vi "Scan_1.vi"(4 "error in":errorcluster, 5 "input main cluster":T2, 7 "Map geometry":T1) -> (0 "error out":errorcluster, 1 "output main cluster":T2)   [LabVIEW 2010]
uses:
  Main_cluster.ctl
  <vilib>/vision/Image Controls.llb/IMAQ Image.ctl
  PI E710 Stage.lvlib
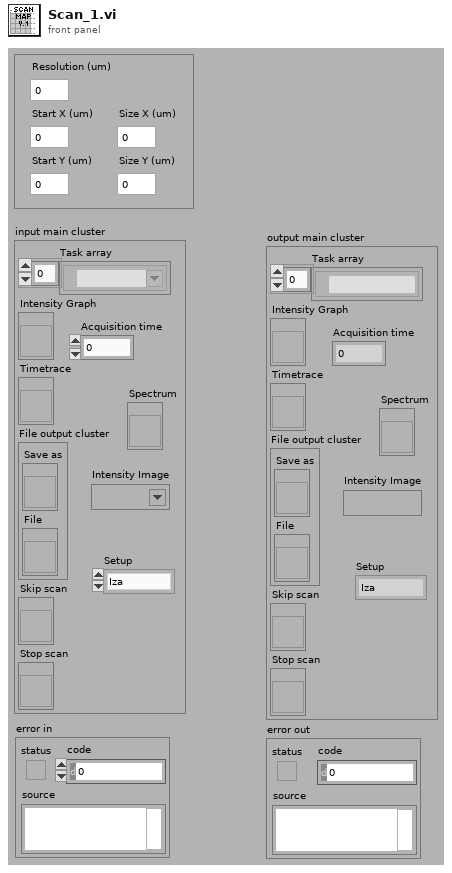
[diagram p1: front panel]
types:
  T1 = cluster{"Size Y (um)":dbl, "Size X (um)":dbl, "Start Y (um)":dbl, "Start X (um)":dbl, "Resolution (um)":dbl}
  T2 = typedef "Main_cluster.ctl" = cluster{"Task array":refnum<k21>[], "Intensity Graph":refnum<vi>, "Timetrace":refnum<vi>, "File output cluster":cluster{"Save as":refnum<vi>, "File":refnum<vi>}, "Skip scan":refnum<vi>, "Stop scan":refnum<vi>, "Acquisition time":dbl, "Setup":enum16{"Iza", "Lukasz"}, "Spectrum":refnum<vi>, "Intensity Image":T3}
  T3 = typedef "IMAQ Image.ctl" = refnum<image>
  T4 = enum16{"open", "replace", "create", "open or create", "replace or create", "replace or create with confirmation"}
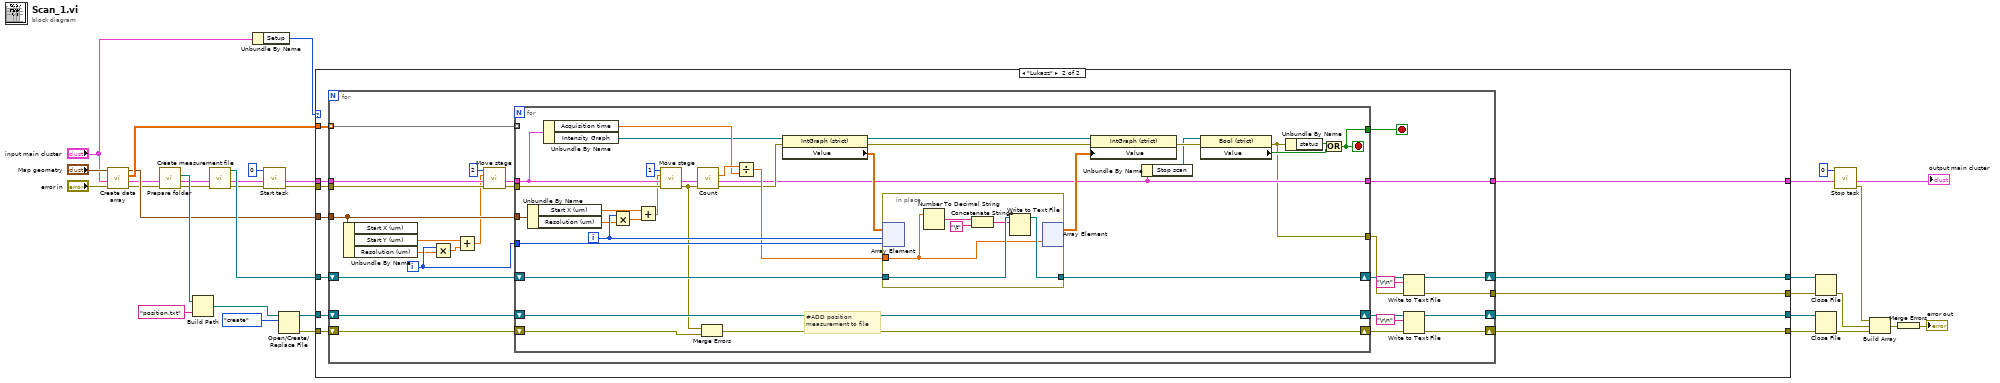
[diagram p0: block diagram]
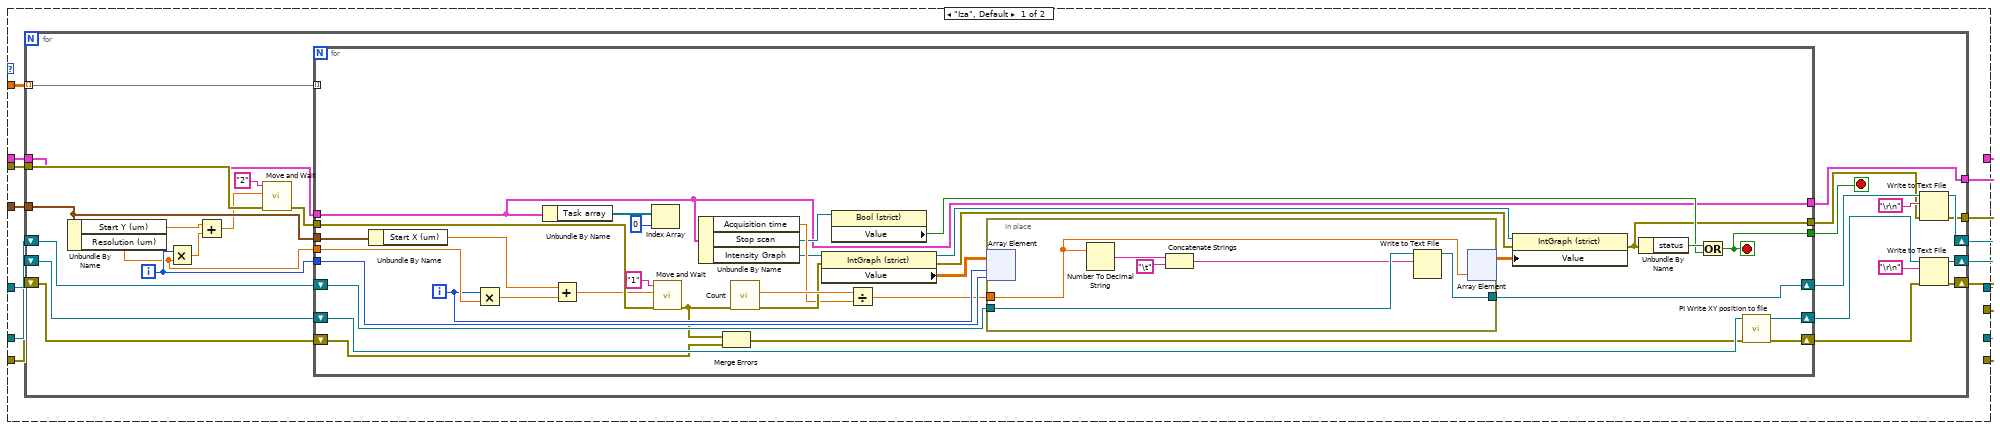
[diagram p2: hidden frame]
diagram:
  n1 = call "Create data array.vi"("error in"="error in", "input main cluster"="input main cluster", "Map geometry"="Map geometry") -> ("error out"=w3:errorcluster, "output main cluster"=w4:T2, "Data array"=w19:dbl[][], "Map geometry out"=w6:T1)  [unwired: 1 in]
  n2 = call "Prepare folder.vi"("error in"=w3, "input main cluster"=w4) -> ("error out"=w8:errorcluster, "output main cluster"=w9:T2, "created path"=w23:path)  [unwired: 3 in]
  n3 = Build Path(base path=w23, name or relative path="position.txt" ("string")) -> (appended path=w30:path)
  n4 = call "Create measurement file.vi"("error in"=w8, "input main cluster"=w9) -> ("error out"=w17:errorcluster, "output main cluster"=w11:T2, "refnum out"=w34:refnum<file>)  [unwired: 3 in]
  n5 = Unbundle By Name("input main cluster") -> ("Setup"=w20:enum16{"Iza", "Lukasz"})
  n6 = call "Start task.vi"("error in"=w17, "input main cluster"=w11, "index"=0) -> ("error out"=w16:errorcluster, "output cluster"=w14:T2)  [unwired: 3 in]
  n7 = Open/Create/Replace File(file path (use dialog)=w30, operation (0:open)=T4."create") -> (refnum out=w29:refnum<file>, error out=w28:errorcluster)  [unwired: 4 in, 1 out]
  n8 = case shown="\"Lukasz\"" w20 {
    tunnel: w16 -> [w46 w124]
    tunnel: w34 -> [w45 w123]
    tunnel: [w44 w122] -> w33
    tunnel: [w43 w121] -> w32
    tunnel: w14 -> [w42 w120]
    tunnel: [w41 w119] -> w18
    tunnel: w19 -> [w40 w118]
    tunnel: w6 -> [w39 w117]
    tunnel: w29 -> [w38 w116]
    tunnel: w28 -> [w37 w115]
    tunnel: [w36 w114] -> w27
    tunnel: [w35 w113] -> w2
    frame "Iza", Default {
      n9 = for {
        tunnel: w46 -> [w72]
        tunnel: [w61] -> w43
        shift-right: [w64] -> w44
        shift-left: w45 -> [w67]
        tunnel: w42 -> [w57]
        tunnel: [w60] -> w41
        tunnel: w39 -> [w58]
        tunnel: w40 -> [w47] mode=indexing
        shift-right: [w52] -> w35
        shift-left: w37 -> [w55]
        shift-right: [w50] -> w36
        shift-left: w38 -> [w56]
        i -> [w68]
        stop <- w66 stop-if-true
        n10 = Unbundle By Name(w58) -> ("Start Y (um)"=w59:dbl, "Resolution (um)"=w48:dbl)
        n11 = Multiply(x=w68, y=w48) -> (x*y=w70:dbl)
        n12 = Add(x=w59, y=w70) -> (x+y=w49:dbl)
        n13 = call "Move and Wait.vi"("error IO"=w72, "Absolute position"=w49, "Axis"="2" ("String")) -> ("error out"=w71:errorcluster)  [unwired: 4 in]
        n14 = for {
          tunnel: [w90] -> w62
          tunnel: w71 -> [w88]
          tunnel: w68 -> [w104]
          tunnel: w48 -> [w102]
          tunnel: [w81] -> w66
          shift-right: [w98] -> w65
          shift-left: w67 -> [w99]
          tunnel: w57 -> [w76]
          tunnel: [w76] -> w60
          tunnel: w58 -> [w85]
          tunnel: w47 -> [_] mode=indexing
          shift-right: [w78] -> w53
          shift-left: w55 -> [w74]
          shift-right: [w79] -> w51
          shift-left: w56 -> [w80]
          i -> [w100]
          stop <- w81 stop-if-true
          n15 = Unbundle By Name(w85) -> ("Start X (um)"=w86:dbl)
          n16 = Multiply(x=w100, y=w102) -> (x*y=w103:dbl)
          n17 = Unbundle By Name(w76) -> ("Task array"=w83:refnum<k21>[])
          n18 = Add(x=w86, y=w103) -> (x+y=w77:dbl)
          n19 = Index Array(array=w83, index=0) -> ()  [unwired: 1 out]
          n20 = call "Move and Wait.vi"("error IO"=w88, "Absolute position"=w77, "Axis"="1" ("String")) -> ("error out"=w73:errorcluster)  [unwired: 4 in]
          n21 = Unbundle By Name(w76) -> ("Acquisition time"=w89:dbl, "Stop scan"=w87:refnum<vi>, "Intensity Graph"=w84:refnum<vi>)
          n22 = Merge Errors(w73, w74) -> (w75:errorcluster)
          n23 = call "Count.vi"("error in"=w73) -> ("error out"=w92:errorcluster, "Counts"=w95:dbl)  [unwired: 4 in, 1 out]
          n24 = property class="IntGraph (strict)"(reference=w84, error in=w92) -> (reference out=w93:refnum<vi>, error out=w91:errorcluster, "Value"=w106:dbl[][])
          n25 = property class="Bool (strict)"(reference=w87) -> ("Value"=w94:bool)  [unwired: 1 in, 2 out]
          n26 = Divide(x=w95, y=w89) -> (x/y=w96:dbl)
          n27 = in-place {
            in-place-border: w96 -> [w109]
            in-place-border: w99 -> [w112]
            in-place-border: [w111] -> w98
            n28 = in-place-array #1(w106, w100, w104) -> ()  [unwired: 1 out]
            n29 = Number To Decimal String(number=w109) -> (decimal integer string=w110:string)  [unwired: 1 in]
            n30 = Concatenate Strings(w110, "\t") -> (w107:string)
            n31 = Write to Text File(file (use dialog)=w112, text=w107) -> (refnum out=w111:refnum<file>)  [unwired: 2 in, 2 out]
            n32 = in-place-array #1(w109) -> (w105:dbl[][])  [unwired: 2 out]
          }
          n33 = property class="IntGraph (strict)"(reference=w93, error in=w91, "Value"=w105) -> (error out=w90:errorcluster)  [unwired: 1 out]
          n34 = Unbundle By Name(w90) -> ("status"=w97:bool)
          n35 = Or(x=w97, y=w94) -> (x .or. y?=w81:bool)
          n36 = call "PI Write XY position to file.vi"("error in"=w75, "refnum in"=w80) -> ("error out"=w78:errorcluster, "refnum out"=w79:refnum<file>)  [unwired: 4 in]
        }
        n37 = Write to Text File(file (use dialog)=w65, text="\r\n", error in=w62) -> (refnum out=w64:refnum<file>, error out=w61:errorcluster)  [unwired: 1 in, 1 out]
        n38 = Write to Text File(file (use dialog)=w51, text="\r\n", error in=w53) -> (refnum out=w50:refnum<file>, error out=w52:errorcluster)  [unwired: 1 in, 1 out]
      }
    }
    frame "Lukasz" {
      n39 = for {
        tunnel: w124 -> [w131]
        tunnel: [w143] -> w121
        shift-right: [w146] -> w122
        shift-left: w123 -> [w149]
        tunnel: w120 -> [w129]
        tunnel: [w142] -> w119
        tunnel: w117 -> [w140]
        tunnel: w118 -> [w139] mode=indexing
        shift-right: [w134] -> w113
        shift-left: w115 -> [w137]
        shift-right: [w132] -> w114
        shift-left: w116 -> [w138]
        i -> [w150]
        stop <- w148 stop-if-true
        n40 = Unbundle By Name(w140) -> ("Start Y (um)"=w141:dbl, "Resolution (um)"=w127:dbl)  [unwired: 1 out]
        n41 = Multiply(x=w150, y=w127) -> (x*y=w151:dbl)
        n42 = Add(x=w141, y=w151) -> (x+y=w125:dbl)
        n43 = call "Move stage.vi"("error in"=w131, "input main cluster"=w129, "position"=w125, "Axis"=2) -> ("error out"=w130:errorcluster, "output main cluster"=w128:T2)  [unwired: 2 in]
        n44 = for {
          tunnel: [w153] -> w144
          tunnel: w130 -> [w161]
          tunnel: w150 -> [w182]
          tunnel: [w166] -> w148
          shift-right: [w178] -> w147
          shift-left: w149 -> [w179]
          tunnel: w128 -> [w160]
          tunnel: [w155] -> w142
          tunnel: w140 -> [w168]
          tunnel: w139 -> [_] mode=indexing
          shift-right: [w164] -> w135
          shift-left: w137 -> [w163]
          shift-right: [w165] -> w133
          shift-left: w138 -> [w165]
          i -> [w180]
          stop <- w166 stop-if-true
          # "#ADD position \nmeasurement to file"
          n45 = Unbundle By Name(w168) -> ("Start X (um)"=w169:dbl, "Resolution (um)"=w159:dbl)
          n46 = Unbundle By Name(w160) -> ("Acquisition time"=w170:dbl, "Intensity Graph"=w167:refnum<vi>)
          n47 = Multiply(x=w180, y=w159) -> (x*y=w181:dbl)
          n48 = Add(x=w169, y=w181) -> (x+y=w158:dbl)
          n49 = call "Move stage.vi"("error in"=w161, "input main cluster"=w160, "position"=w158, "Axis"=1) -> ("error out"=w162:errorcluster, "output main cluster"=w156:T2)  [unwired: 2 in]
          n50 = call "Count.vi"("error in"=w162, "input cluster"=w156) -> ("error out"=w172:errorcluster, "output cluster"=w155:T2, "Counts"=w175:dbl)  [unwired: 3 in]
          n51 = Merge Errors(w162, w163) -> (w164:errorcluster)
          n52 = Divide(x=w175, y=w170) -> (x/y=w176:dbl)
          n53 = property class="IntGraph (strict)"(reference=w167, error in=w172) -> (reference out=w173:refnum<vi>, error out=w171:errorcluster, "Value"=w184:dbl[][])
          n54 = in-place {
            in-place-border: w176 -> [w187]
            in-place-border: w179 -> [w190]
            in-place-border: [w189] -> w178
            n55 = in-place-array #2(w184, w180, w182) -> ()  [unwired: 1 out]
            n56 = Number To Decimal String(number=w187) -> (decimal integer string=w188:string)  [unwired: 1 in]
            n57 = Concatenate Strings(w188, "\t") -> (w185:string)
            n58 = Write to Text File(file (use dialog)=w190, text=w185) -> (refnum out=w189:refnum<file>)  [unwired: 2 in, 2 out]
            n59 = in-place-array #2(w187) -> (w183:dbl[][])  [unwired: 2 out]
          }
          n60 = property class="IntGraph (strict)"(reference=w173, error in=w171, "Value"=w183) -> (error out=w154:errorcluster)  [unwired: 1 out]
          n61 = Unbundle By Name(w155) -> ("Stop scan"=w152:refnum<vi>)
          n62 = property class="Bool (strict)"(reference=w152, error in=w154) -> (error out=w153:errorcluster, "Value"=w174:bool)  [unwired: 1 out]
          n63 = Unbundle By Name(w153) -> ("status"=w177:bool)
          n64 = Or(x=w177, y=w174) -> (x .or. y?=w166:bool)
        }
        n65 = Write to Text File(file (use dialog)=w147, text="\r\n", error in=w144) -> (refnum out=w146:refnum<file>, error out=w143:errorcluster)  [unwired: 1 in, 1 out]
        n66 = Write to Text File(file (use dialog)=w133, text="\r\n", error in=w135) -> (refnum out=w132:refnum<file>, error out=w134:errorcluster)  [unwired: 1 in, 1 out]
      }
    }
  }
  n67 = Close File(refnum=w33, error in=w32) -> (error out=w10:errorcluster)  [unwired: 1 out]
  n68 = Close File(refnum=w27, error in=w2) -> (error out=w25:errorcluster)  [unwired: 1 out]
  n69 = call "Stop task.vi"("input main cluster"=w18, "index"=0) -> ("error out"=w1:errorcluster, "output main cluster"=→"output main cluster":T2)  [unwired: 4 in]
  n70 = Build Array(w1, w10, w25) -> (w21:errorcluster[])
  n71 = Merge Errors(w21) -> (→"error out":errorcluster)
